vi "PH_AxisGUI_BaseClass.Message Box.vi"(1 "String":string) -> (0 "OK?":bool)   [LabVIEW 2014, in "PH_AxisGUI_BaseClass.lvlib"]
uses:
  PH_AxisGUI_BaseClass.lvlib
panel:
  in  "Cancel":bool
  in  "Ok":bool
  out "Message":string
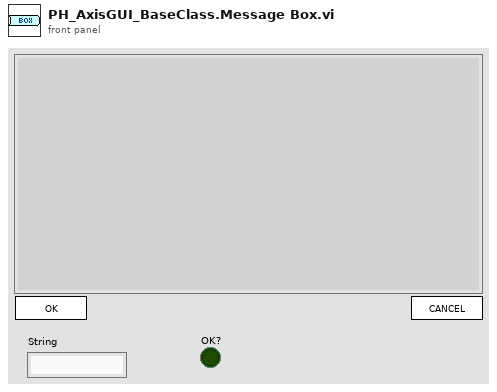
[diagram p1: front panel]
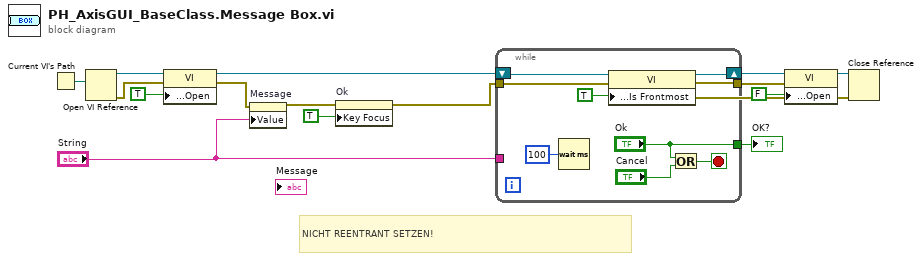
[diagram p0: block diagram]
diagram:
  # "NICHT REENTRANT SETZEN!"
  n1 = Current VI's Path() -> (path=w15:path)
  n2 = Open VI Reference(vi path=w15) -> (vi reference=w13:refnum<vi>, error out=w5:errorcluster)  [unwired: 5 in]
  n3 = property class="VI"(reference=w13, error in=w5, "Front Panel Window:Open"=TRUE) -> (reference out=w14:refnum<vi>, error out=w11:errorcluster)
  n4 = property on="Message" class="Str"(error in=w11, "Value"="String") -> (error out=w3:errorcluster)  [unwired: 1 in, 1 out]
  n5 = property on="Ok" class="Bool"(error in=w3, "Key Focus"=TRUE) -> (error out=w1:errorcluster)  [unwired: 1 in, 1 out]
  n6 = while {
    tunnel: ["Ok"] -> w16
    tunnel: "String" -> [_]
    shift-right: [w20] -> w9
    shift-left: w14 -> [w21]
    tunnel: w1 -> [w17]
    tunnel: [w19] -> w8
    stop <- w23 stop-if-true
    n7 = Wait (ms)(milliseconds to wait=u32 100) -> ()  [unwired: 1 out]
    n8 = property class="VI"(reference=w21, error in=w17, "Front Panel Window:Is Frontmost"=TRUE) -> (reference out=w20:refnum<vi>, error out=w19:errorcluster)
    n9 = Or(x="Ok", y="Cancel") -> (x .or. y?=w23:bool)
  }
  "OK?" <- w16
  n10 = property class="VI"(reference=w9, error in=w8, "Front Panel Window:Open"=FALSE) -> (reference out=w6:refnum<vi>, error out=w7:errorcluster)
  n11 = Close Reference(reference=w6, error in (no error)=w7) -> ()  [unwired: 1 out]
